vi "INSERT PPMS4 (example).vi"() -> ()   [LabVIEW 2019, in "LV-Data.PGSQL.lvclass"]
uses:
  LV-Data.PGSQL.lvclass
panel:
  in  "milliseconds to wait":u32
  out "Written":i32
  in  "rows per insert":i32=50
  in  "stop":bool
  in  "Boolean":bool=TRUE
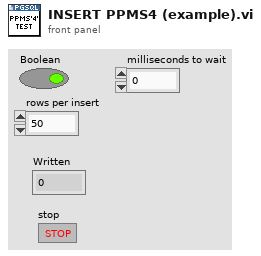
[diagram p1: front panel]
types:
  T1 = cluster{string, string, "Boolean":bool, i32, dbl, dbl, dbl[]}
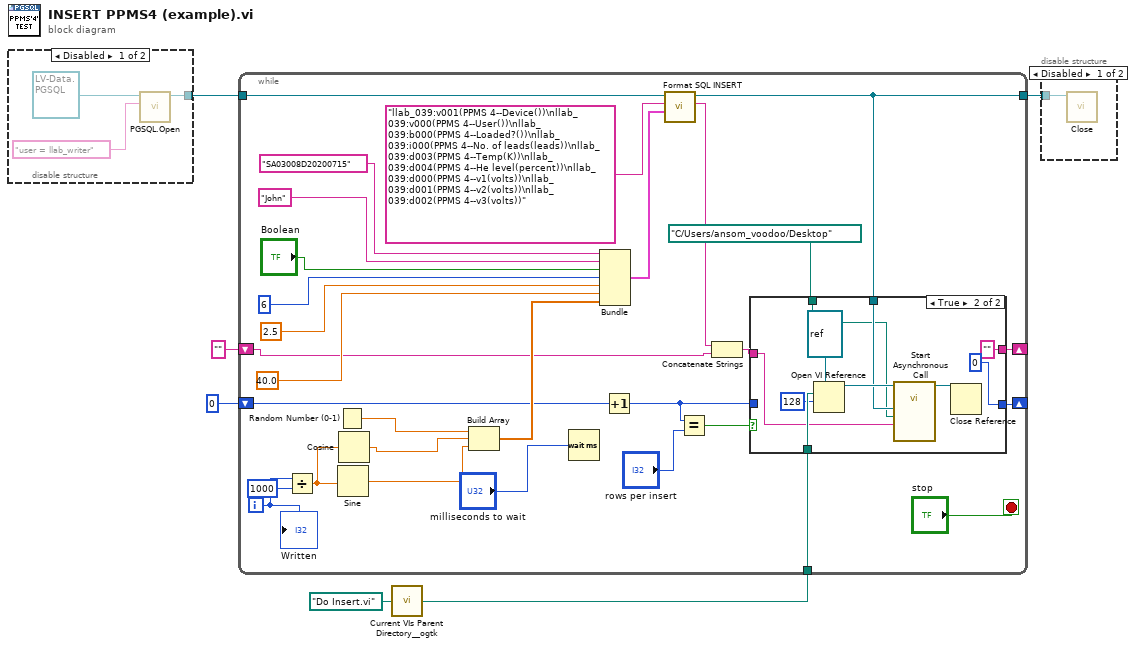
[diagram p0: block diagram]
diagram:
  n1 = disable-structure shown="Disabled" {
    disable-tunnel: [w7 _] -> w2
    frame Disabled {
      n2 = call "PGSQL.Open.vi"("Connection String"="user = llab_writer", "Data.PG in"=refnum<class "LV-Data.PGSQL.lvclass"> refnum ("Database.PG.lvclass")) -> ("Data.PG out"=w7:refnum<class "LV-Data.PGSQL.lvclass">)  [unwired: 8 in, 1 out]
    }
    frame Enabled {
    }
  }
  n3 = call <userlib>:"Current VIs Parent Directory__ogtk.vi"("Relative path (.)"=path "Do Insert.vi") -> ("Parent Directory (+ Relative)"=w3:path)  [unwired: 4 in]
  n4 = while {
    tunnel: w2 -> [w11]
    shift-right: [w22] -> _
    shift-left: 0 -> [w27]
    tunnel: w3 -> [w21]
    shift-right: [w15] -> _
    shift-left: "" -> [w14]
    tunnel: [w12] -> w1
    i -> [w38]
    stop <- "stop" stop-if-true
    n5 = Divide(x=w38, y=1000) -> (x/y=w20:dbl)
    n6 = Random Number (0-1)() -> (number: 0 to 1=w36:dbl)
    n7 = Sine(x=w20) -> (sin(x)=w35:dbl)
    n8 = Cosine(x=w20) -> (cos(x)=w19:dbl)
    n9 = Build Array(w36, w19, w35) -> (w28:dbl[])
    n10 = Wait (ms)(milliseconds to wait="milliseconds to wait") -> ()  [unwired: 1 out]
    n11 = Bundle("SA03008D20200715", "John", "Boolean"="Boolean", 6, 2.5, 40.0, w28) -> (w13:T1)  [unwired: 1 in]
    n12 = Increment(x=w27) -> (x+1=w24:i32)
    n13 = call "Format SQL INSERT.vi"("Data"=w13, "Path(s)"="llab_039:v001(PPMS 4--Device())\nllab_039:v000(PPMS 4--User())\nllab_039:b000(PPMS 4--Loaded?())\nllab_039:i000(PPMS 4--No. of leads(leads))\nllab_039:d003(PPMS 4--Temp(K))\nllab_039:d004(PPMS 4--He level(percent))\nllab_039:d000(PPMS 4--v1(volts))\nllab_039:d001(PPMS 4--v2(volts))\nllab_039:d002(PPMS 4--v3(volts))", "LV-Data.PGSQL in"=w11) -> ("Formatted Insert"=w17:string, "LV-Data.PGSQL out"=w12:refnum<class "LV-Data.PGSQL.lvclass">)  [unwired: 5 in, 2 out]
    n14 = Equal?(x=w24, y="rows per insert") -> (x = y?=w25:bool)
    n15 = Concatenate Strings(w17, w14) -> (w16:string)
    n16 = case shown="True" w25 {
      tunnel: w24 -> [w41 _]
      tunnel: w16 -> [w40 w43]
      tunnel: path "C:/Users/ansom_voodoo/Desktop" ("backup storage folder") -> [_ w45]
      tunnel: w12 -> [_ w46]
      tunnel: [w41 0] -> w22
      tunnel: w21 -> [_ w50]
      tunnel: [w40 ""] -> w15
      frame False {
      }
      frame True {
        n17 = Open VI Reference(type specifier VI Refnum (for type only)=refnum<vi> refnum, vi path=w50, options=128) -> (vi reference=w47:refnum<vi>)  [unwired: 3 in, 1 out]
        n18 = call-by-ref "Start Asynchronous Call"(reference=w47, "Formatted Insert"=w43, "backup storage folder"=w45, "Data.PG in"=w46) -> (reference out=w44:refnum<vi>)  [unwired: 7 in, 4 out]
        n19 = Close Reference(reference=w44) -> ()  [unwired: 1 in, 1 out]
      }
    }
    "Written" <- w38
  }
  n20 = disable-structure shown="Disabled" {
    disable-tunnel: w1 -> [w52 _]
    frame Disabled {
      n21 = call-dynamic "Close.vi"("Data.PG in"=w52) -> ()  [unwired: 9 in, 2 out]
    }
    frame Enabled {
    }
  }
